vi "mod_Generate guard and sync bits.vi"(0 "# Guard Bits":i32=2, 5 "# Sync Bits":i32=20, 11 "error in (no error)":errorcluster) -> (4 "Guard Bits":i8[](array[numeric]), 6 "Sync Bits":i8[](array[numeric]), 15 "error out":errorcluster)   [LabVIEW 2020, in "niDMT.lvlib"]
uses:
  <vilib>/addons/Modulation/niDMT.lvlib
  <vilib>/addons/Modulation/Digital/Support/Common/Validators/mod_Generate Bits Validate.vi
  <vilib>/addons/Modulation/Digital/General/subVIs/mod_Generate Bits Pattern.vi
  <vilib>/addons/Modulation/Analog/support/mod_Set Error Source.vi
  <vilib>/addons/Modulation/Digital/General/subVIs/mod_Generate Bits PN Sequence.vi
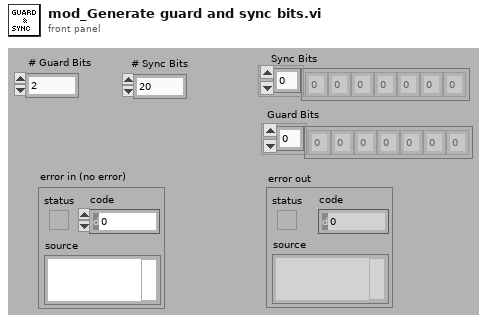
[diagram p1: front panel]
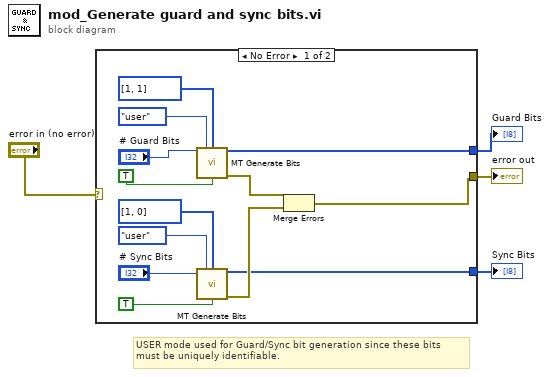
[diagram p0: block diagram]
diagram:
  # "USER mode used for Guard/Sync bit generation since these bits\nmust be uniquely identifiable."
  n1 = case shown="No Error" "error in (no error)" {
    selector: "error in (no error)" -> [_ w18]
    tunnel: [w10 w18] -> w3
    tunnel: [w6 _] -> w2
    tunnel: [w5 _] -> w1
    frame No Error {
      n2 = call <vilib>:"MT Generate Bits.vi"("total bits (128)"="# Guard Bits", "mode (PN)"=enum16{"PN", "pattern", "user"}."user" ("Mode (PN)"), "user base bit pattern"=i8[] [1, 1] ("User Base Bit Pattern"), "reset? (T)"=TRUE ("Reset? (T)")) -> ("output bit stream"=w6:i8[], "error out"=w12:errorcluster)  [unwired: 4 in, 6 out]
      n3 = call <vilib>:"MT Generate Bits.vi"("total bits (128)"="# Sync Bits", "mode (PN)"=enum16{"PN", "pattern", "user"}."user" ("Mode (PN)"), "user base bit pattern"=i8[] [1, 0] ("User Base Bit Pattern"), "reset? (T)"=TRUE ("Reset? (T)")) -> ("output bit stream"=w5:i8[], "error out"=w11:errorcluster)  [unwired: 4 in, 6 out]
      n4 = Merge Errors(w12, w11) -> (w10:errorcluster)
    }
    frame Error {
    }
  }
  "error out" <- w3
  "Guard Bits" <- w2
  "Sync Bits" <- w1
